vi "Gear Mech Controller.vi"(8 "error in":errorcluster) -> ()   [LabVIEW 2016]
doc: "This VI executes continuously carrying out the current operation and responding to updates or new operations. It will often contain the timing or control code that is difficult to place directly in TeleOp. This VI generally opens all sensors and motors and isolates the rest of the robot code from knowing how the operations are carried out."
uses:
  <vilib>/Rock Robotics/WPI/ThirdParty/CanMotor/TalonSRX/WPI_CANTalonSRX_GlobalStatus.ctl
  Shared/PID Settings.ctl
  Gear Mech Setpoints.ctl
  Gear Mech Operations.ctl
  <vilib>/Rock Robotics/WPI/ThirdParty/CanMotor/TalonSRX/WPI_CANTalonSRX_APIControlMode.ctl
  <vilib>/Rock Robotics/WPI/ThirdParty/CanMotor/TalonSRX/WPI_CANTalonSRX_APIFeedbackSelect.ctl
  <vilib>/Rock Robotics/Network Tables/NT Write Boolean.vi
panel:
  in  "Full Up Position":dbl=600.0
  in  "Boolean":bool
  in  "Shooter PID":T1={"D"=0.01, "F"=0.0, "RR"=0.0, "IZ"=0.0, "P"=3.0, "I"=0.0}
  in  "Down Position":dbl=345.0
  in  "Up Position":dbl=560.0
  in  "In Speed":dbl=0.5
  in  "Out Speed":dbl=-0.5
  out "Talon SRX Status":T2
  out "Current\nCmd":string
  # "Tip: It may be helpful to observe inputs and sensor values.\nYou may also want to display tuning or debugging controls."
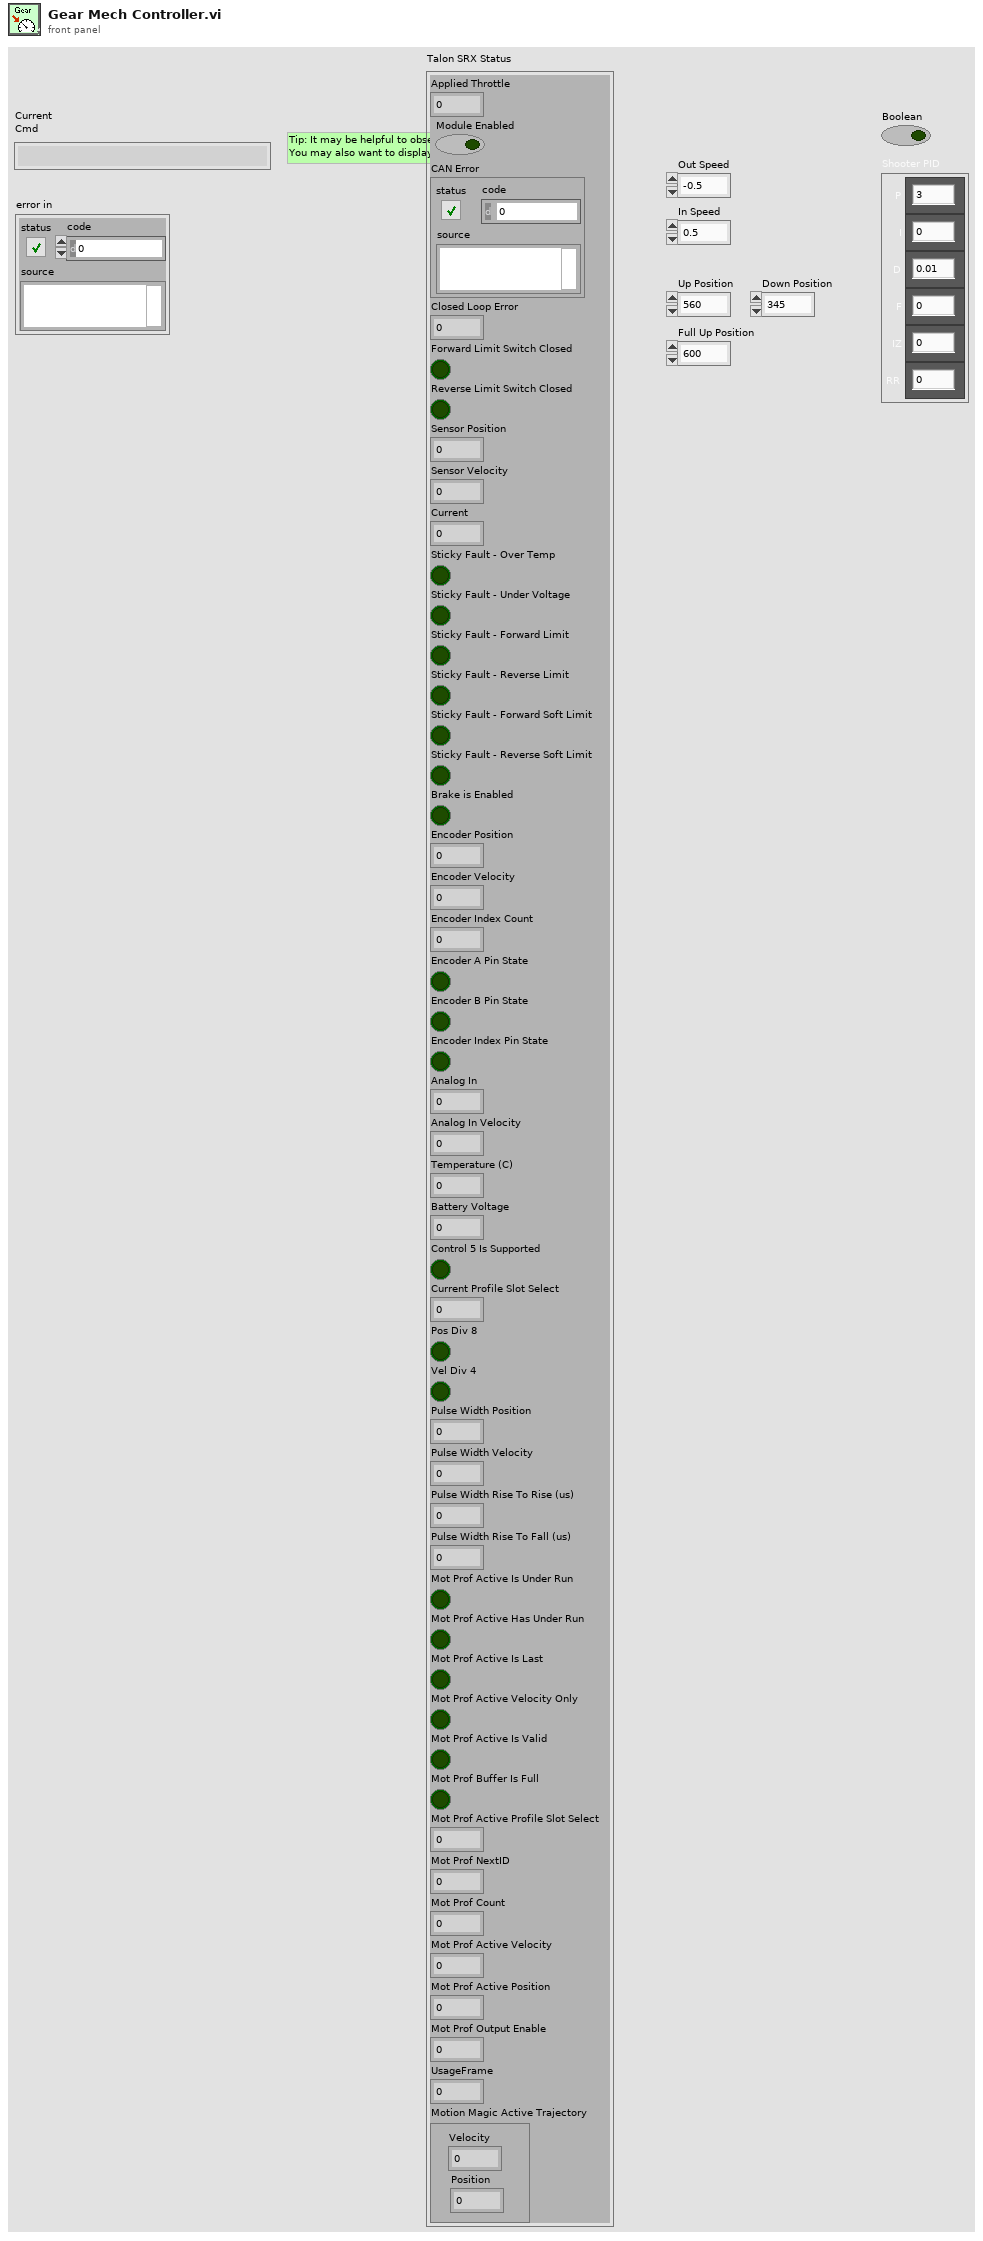
[diagram p1: front panel]
types:
  T1 = typedef "PID Settings.ctl" = cluster{"D":dbl, "F":dbl, "RR":dbl, "IZ":dbl, "P":dbl, "I":dbl}
  T2 = typedef "WPI_CANTalonSRX_GlobalStatus.ctl" = cluster{"Applied Throttle":dbl, "Module Enabled":bool, "CAN Error":errorcluster, "Closed Loop Error":dbl, "Forward Limit Switch Closed":bool, "Reverse Limit Switch Closed":bool, "Sensor Position":dbl, "Sensor Velocity":dbl, "Current":dbl, "Sticky Fault - Over Temp":bool, "Sticky Fault - Under Voltage":bool, "Sticky Fault - Forward Limit":bool, "Sticky Fault - Reverse Limit":bool, "Sticky Fault - Forward Soft Limit":bool, "Sticky Fault - Reverse Soft Limit":bool, "Brake is Enabled":bool, "Encoder Position":dbl, "Encoder Velocity":dbl, "Encoder Index Count":dbl, "Encoder A Pin State":bool, "Encoder B Pin State":bool, "Encoder Index Pin State":bool, "Analog In":dbl, "Analog In Velocity":dbl, "Temperature (C)":dbl, "Battery Voltage":dbl, "Control 5 Is Supported":bool, "Current Profile Slot Select":dbl, "Pos Div 8":bool, "Vel Div 4":bool, "Pulse Width Position":i32, "Pulse Width Velocity":i32, "Pulse Width Rise To Rise (us)":i32, "Pulse Width Rise To Fall (us)":i32, "Mot Prof Active Is Under Run":bool, "Mot Prof Active Has Under Run":bool, "Mot Prof Active Is Last":bool, "Mot Prof Active Velocity Only":bool, "Mot Prof Active Is Valid":bool, "Mot Prof Buffer Is Full":bool, "Mot Prof Active Profile Slot Select":i32, "Mot Prof NextID":i32, "Mot Prof Count":i32, "Mot Prof Active Velocity":dbl, "Mot Prof Active Position":dbl, "Mot Prof Output Enable":i32, "UsageFrame":u32, "Motion Magic Active Trajectory":cluster{"Velocity":dbl, "Position":dbl}}
  T3 = typedef "WPI_CANTalonSRX_APIControlMode.ctl" = enum8{"Percent VBus", "Speed", "Position", "Slave", "Unchanged / Invalid", "Voltage Compensation", "Current", "Motion Profile", "Motion Magic"}
  T4 = typedef "WPI_CANTalonSRX_APIFeedbackSelect.ctl" = enum16{"Digital Quadrature Encoder", "Analog Potentiometer", "Analog Encoder", "Count on Quad-A (Rising-Edge)", "Count on Quad-A (Falling-Edge)", "CTR Magnetic Enc (Absolute)", "CTR Magnetic Enc (Relative)", "Pulse Width"}
  T5 = typedef "Gear Mech Setpoints.ctl" = cluster{"Operation":T6, "Setpoint":dbl, "Duration":dbl}
  T6 = typedef "Gear Mech Operations.ctl" = enum16{"Reserve", "Read Current", "Immediate", "Release", "Grab", "Up", "Down", "Full Up"}
  T7 = typedef "WPI_MotorControlDeviceRef.ctl" = cluster{"DeviceStatus":errorcluster, "Type":T8, "PWM":cluster{"PWM Channel":T9, "DeadBand":T10}, "CAN":cluster{"Device Number":u8, "SetOutput VI Ref":variant, "GetOutput VI Ref":variant, "Enable VI Ref":variant, "Disable VI Ref":variant, "Data":variant}, "Invert":bool}
  T8 = typedef "WPI_MotorControlType.ctl" = enum16{"PWM", "CAN"}
  T9 = typedef "FPGA_DIOPWMChannel.ctl" = enum8{"PWM 0", "PWM 1", "PWM 2", "PWM 3", "PWM 4", "PWM 5", "PWM 6", "PWM 7", "PWM 8", "PWM 9", "PWM MXP 0", "PWM MXP 1", "PWM MXP 2", "PWM MXP 3", "PWM MXP 4", "PWM MXP 5", "PWM MXP 6", "PWM MXP 7", "PWM MXP 8", "PWM MXP 9", "Invalid"}
  T10 = typedef "WPI_PWMDeadband.ctl" = cluster{"Name":string, "maxPositivePwm":i32, "minPositivePwm":i32, "centerPwm":i32, "maxNegativePwm":i32, "minNegativePwm":i32, "angularRange":u16}
  T11 = typedef "Command Status Info.ctl" = cluster{"Name":string, "Status":T12, "notifier out":T13}
  T12 = typedef "Completion Status.ctl" = enum16{"Successful", "Aborted", "Incomplete"}
  T13 = typedef "Completion Notifier.ctl" = refnum<notifier>
  T14 = cluster{"Default Command":T5, "Command Timing":cluster{"Start Time (ms)":u32, "Iterations":i32}, "Command Arguments":cluster{"Command Info":T11, "Description":string, "Default Command":T5, "notifier out":refnum<notifier>, "Subsystem Name":string}}
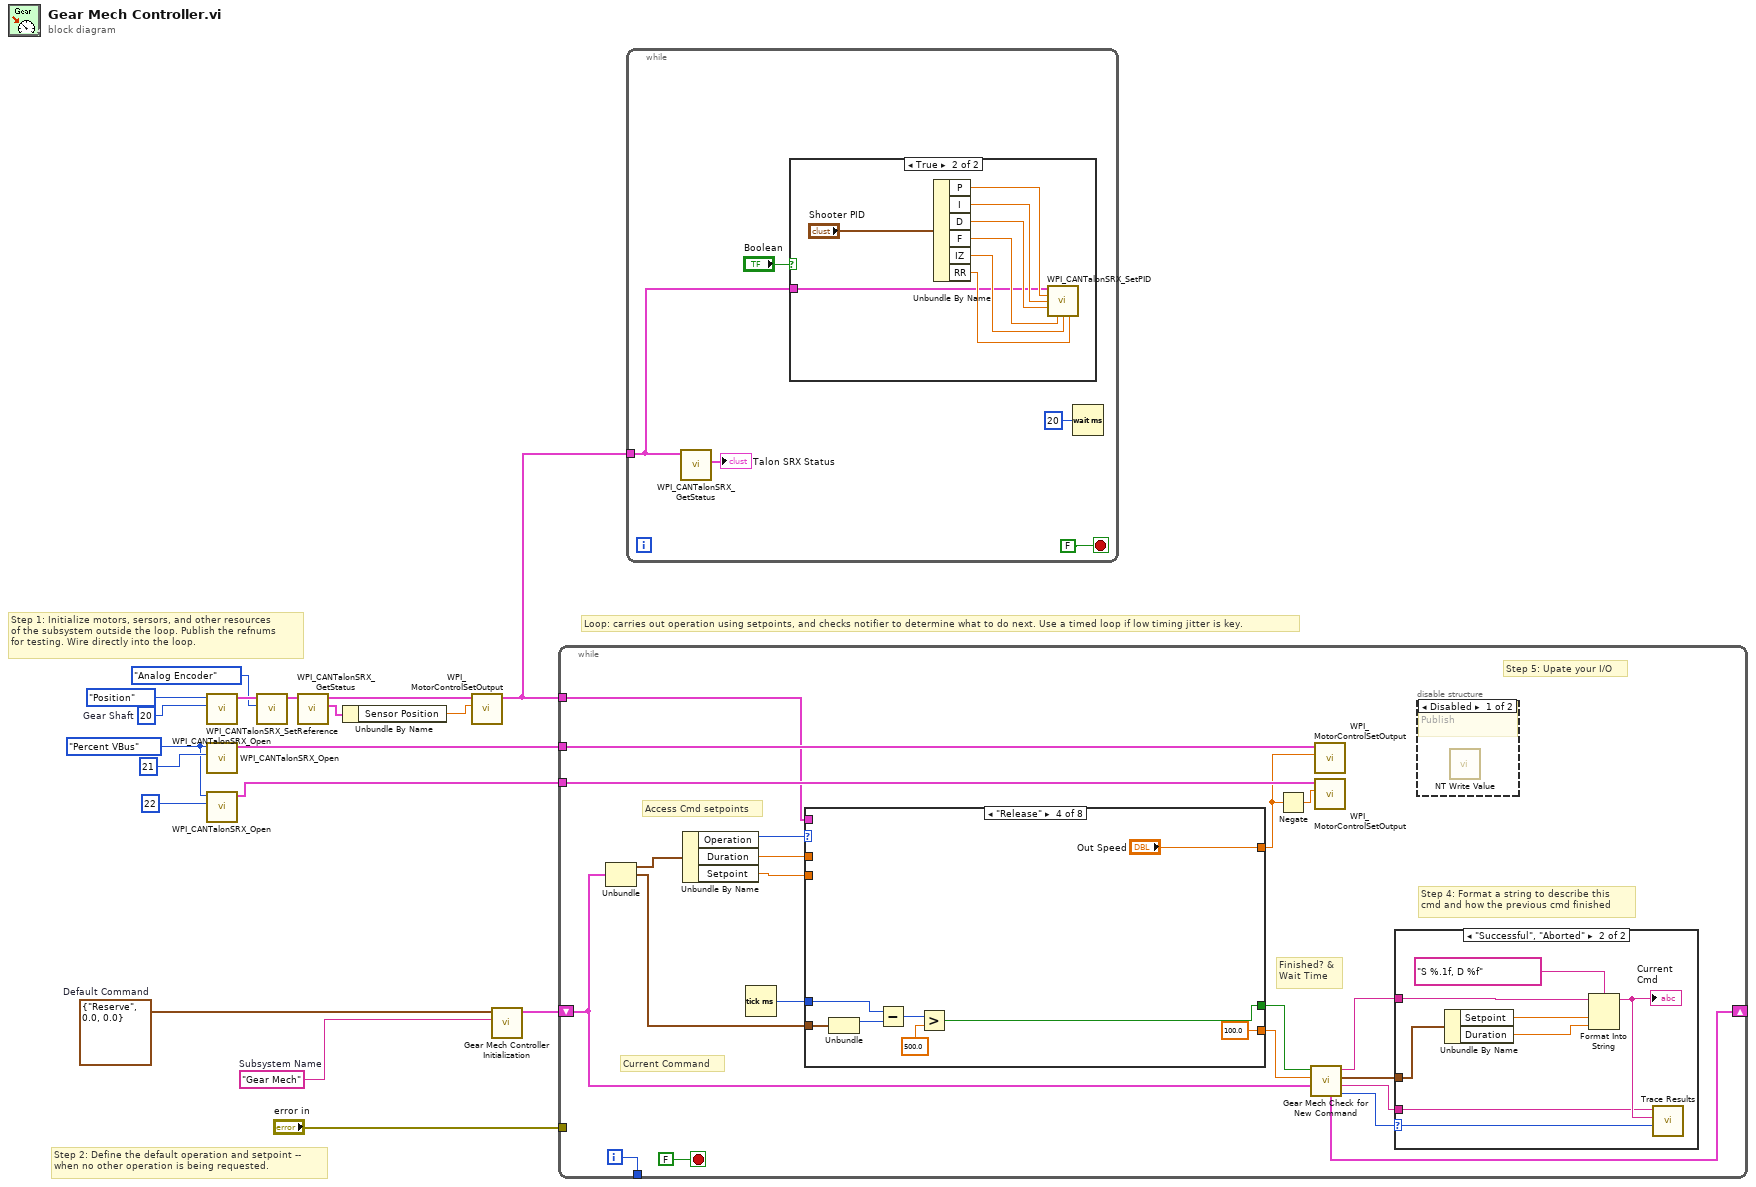
[diagram p0: block diagram]
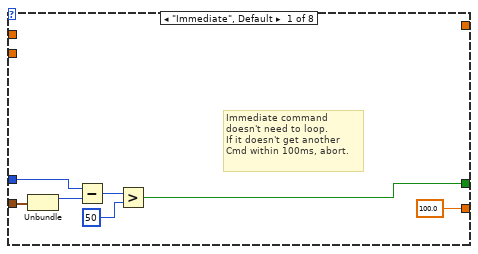
[diagram p5: hidden frame]
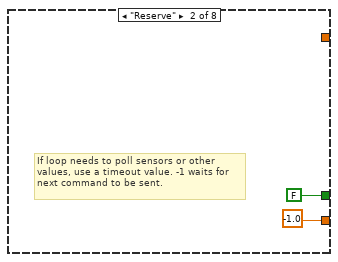
[diagram p6: hidden frame]
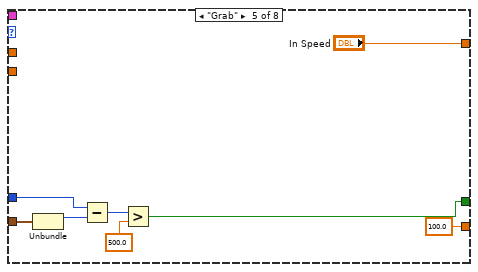
[diagram p8: hidden frame]
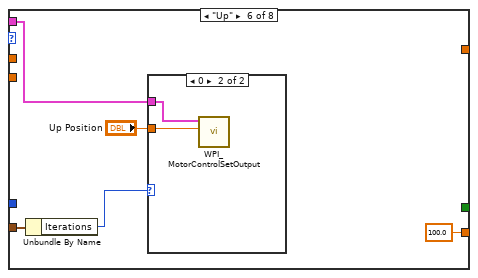
[diagram p9: hidden frame]
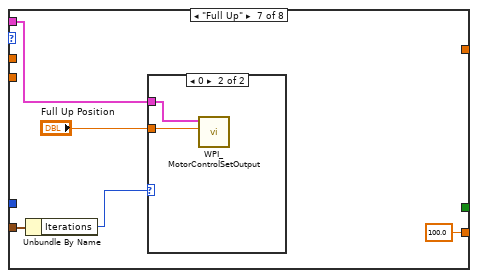
[diagram p11: hidden frame]
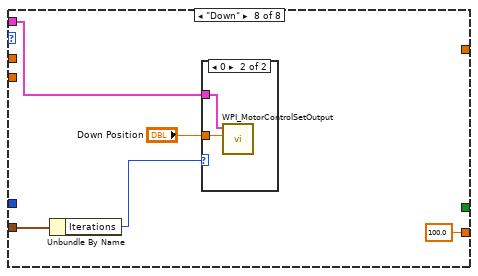
[diagram p13: hidden frame]
diagram:
  w7 = WPI_CANTalonSRX_APIControlMode."Percent VBus" ("Control Mode")
  w13 = u8 20  # Gear Shaft
  w15 = T5 {"Operation"=enum."Reserve", "Setpoint"=0.0, "Duration"=0.0}  # Default Command
  w16 = "Gear Mech"  # Subsystem Name
  # "Step 2: Define the default operation and setpoint --\nwhen no other operation is being requested."
  # "Step 1: Initialize motors, sersors, and other resources\nof the subsystem outside the loop. Publish the refnums\nfor testing. Wire directly into the loop."
  # "Loop: carries out operation using setpoints, and checks notifier to determine what to do next. Use a timed loop if low timing jitter is key."
  n1 = call <vilib>:"WPI_CANTalonSRX_Open.vi"("Device Number"=w13, "Control Mode"=WPI_CANTalonSRX_APIControlMode."Position") -> ("CAN Talon SRX Ref"=w12:T7)  [unwired: 8 in, 1 out]
  n2 = call <vilib>:"WPI_CANTalonSRX_Open.vi"("Device Number"=u8 21, "Control Mode"=w7) -> ("CAN Talon SRX Ref"=w10:T7)  [unwired: 8 in, 1 out]
  n3 = call <vilib>:"WPI_CANTalonSRX_Open.vi"("Device Number"=u8 22, "Control Mode"=w7) -> ("CAN Talon SRX Ref"=w6:T7)  [unwired: 8 in, 1 out]
  n4 = call <vilib>:"WPI_CANTalonSRX_SetReference.vi"("Feedback Reference"=WPI_CANTalonSRX_APIFeedbackSelect."Analog Encoder", "CAN Talon SRX Ref"=w12) -> ("CAN Talon SRX Ref"=w5:T7)  [unwired: 8 in, 1 out]
  n5 = call <vilib>:"WPI_CANTalonSRX_GetStatus.vi"("CAN Talon SRX Ref"=w5) -> ("Talon SRX Status"=w4:T2, "CAN Talon SRX Ref"=w3:T7)  [unwired: 8 in, 1 out]
  n6 = Unbundle By Name(w4) -> ("Sensor Position"=w1:dbl)
  n7 = call <vilib>:"WPI_MotorControlSetOutput.vi"("Output"=w1, "MotorControlDevRef"=w3) -> ("MotorControlDevRef"=w2:T7)  [unwired: 7 in, 2 out]
  n8 = call "Gear Mech Controller Initialization.vi"("Subsystem Name"=w16, "Default Command"=w15) -> ("Command Info"=w17:T14)  [unwired: 9 in]
  n9 = while {
    shift-right: [w30] -> _
    shift-left: w17 -> [w31]
    tunnel: [w38] -> _
    tunnel: "error in" -> [_]
    tunnel: w2 -> [w19]
    tunnel: w10 -> [w23]
    tunnel: w6 -> [w22]
    i -> [w38]
    stop <- FALSE stop-if-true
    # "Step 5: Upate your I/O"
    # "Step 4: Format a string to describe this\ncmd and how the previous cmd finished"
    # "Current Command"
    # "Access Cmd setpoints"
    # "Finished? &\nWait Time"
    n10 = Unbundle(w31) -> ("Default Command"=w37:T5, "Command Timing"=w33:cluster{"Start Time (ms)":u32, "Iterations":i32})  [unwired: 1 out]
    n11 = Unbundle By Name(w37) -> ("Operation"=w36:T6, "Duration"=w35:dbl, "Setpoint"=w32:dbl)
    n12 = Tick Count (ms)() -> (millisecond timer value=w34:u32)
    n13 = case shown="\"Release\"" w36 {
      tunnel: [100.0 -1.0 _ 100.0 100.0 100.0 100.0 100.0] -> w28
      tunnel: [w48 FALSE ("ignore previous (F)") _ w58 w66 _ _ _] -> w29
      tunnel: w33 -> [w50 _ _ w60 w68 w76 w83 w89]
      tunnel: w35 -> [_ _ _ _ _ _ _ _]
      tunnel: w34 -> [w49 _ _ w59 w67 _ _ _]
      tunnel: w32 -> [_ _ _ _ _ _ _ _]
      tunnel: [_ _ _ "Out Speed" "In Speed" _ _ _] -> w21
      tunnel: w19 -> [_ _ _ _ _ w74 w81 w87]
      frame "Immediate", Default {
        # "Immediate command\ndoesn't need to loop.\nIf it doesn't get another\nCmd within 100ms, abort."
        n14 = Unbundle(w50) -> ("Start Time (ms)"=w53:u32)  [unwired: 1 out]
        n15 = Subtract(x=w49, y=w53) -> (x-y=w52:u32)
        n16 = Greater?(x=w52, y=u8 50 ("Left Motor")) -> (0:w48:bool)
      }
      frame "Reserve" {
        # "If loop needs to poll sensors or other\nvalues, use a timeout value. -1 waits for\nnext command to be sent."
      }
      frame "Read Current" {
      }
      frame "Release" {
        n17 = Unbundle(w60) -> ("Start Time (ms)"=w61:u32)  [unwired: 1 out]
        n18 = Subtract(x=w59, y=w61) -> (x-y=w63:u32)
        n19 = Greater?(x=w63, y=500.0 ("Out Time")) -> (0:w58:bool)
      }
      frame "Grab" {
        n20 = Unbundle(w68) -> ("Start Time (ms)"=w69:u32)  [unwired: 1 out]
        n21 = Subtract(x=w67, y=w69) -> (x-y=w71:u32)
        n22 = Greater?(x=w71, y=500.0 ("In Time")) -> (0:w66:bool)
      }
      frame "Up" {
        n23 = Unbundle By Name(w76) -> ("Iterations"=w75:i32)
        n24 = case shown="0" w75 {
          tunnel: w74 -> [_ w79]
          tunnel: "Up Position" -> [_ w78]
          frame Default {
          }
          frame 0 {
            n25 = call <vilib>:"WPI_MotorControlSetOutput.vi"("Output"=w78, "MotorControlDevRef"=w79) -> ()  [unwired: 7 in, 3 out]
          }
        }
      }
      frame "Full Up" {
        n26 = Unbundle By Name(w83) -> ("Iterations"=w82:i32)
        n27 = case shown="0" w82 {
          tunnel: w81 -> [_ w86]
          tunnel: "Full Up Position" -> [_ w85]
          frame Default {
          }
          frame 0 {
            n28 = call <vilib>:"WPI_MotorControlSetOutput.vi"("Output"=w85, "MotorControlDevRef"=w86) -> ()  [unwired: 7 in, 3 out]
          }
        }
      }
      frame "Down" {
        n29 = Unbundle By Name(w89) -> ("Iterations"=w90:i32)
        n30 = case shown="0" w90 {
          tunnel: "Down Position" -> [_ w93]
          tunnel: w87 -> [_ w92]
          frame Default {
          }
          frame 0 {
            n31 = call <vilib>:"WPI_MotorControlSetOutput.vi"("Output"=w93, "MotorControlDevRef"=w92) -> ()  [unwired: 7 in, 3 out]
          }
        }
      }
    }
    n32 = Negate(x=w21) -> (-x=w20:dbl)
    n33 = call "Gear Mech Check for New Command.vi"("Current Command"=w31, "Wait time (ms)"=w28, "Finished?"=w29) -> ("Completion"=w24:T12, "Subsystem Name"=w25:string, "Current Command"=w26:T5, "Initial Trace String"=w27:string, "NextCommand"=w30:T14)  [unwired: 4 in]
    n34 = call <vilib>:"WPI_MotorControlSetOutput.vi"("Output"=w21, "MotorControlDevRef"=w23) -> ()  [unwired: 7 in, 3 out]
    n35 = call <vilib>:"WPI_MotorControlSetOutput.vi"("Output"=w20, "MotorControlDevRef"=w22) -> ()  [unwired: 7 in, 3 out]
    n36 = case shown="\"Successful\", \"Aborted\"" w24 {
      selector: w24 -> [_ w47]
      tunnel: w27 -> [_ w43]
      tunnel: w26 -> [_ w44]
      tunnel: w25 -> [_ w40]
      frame "Incomplete", Default {
        # "Continuing current command"
      }
      frame "Successful", "Aborted" {
        # "Report and setup for next command"
        n37 = Unbundle By Name(w44) -> ("Setpoint"=w46:dbl, "Duration"=w41:dbl)
        n38 = Format Into String(format string="S %.1f, D %f", initial string=w43, w46, w41) -> (resulting string=w42:string)  [unwired: 1 in, 1 out]
        "Current\nCmd" <- w42
        n39 = call <vilib>:"Trace Results.vi"("Status of previous command"=w47, "Description"=w42, "Subsystem"=w40) -> ()  [unwired: 9 in]
      }
    }
    n40 = disable-structure shown="Disabled" {
      frame Disabled {
        # "Publish"
        n41 = call-poly <vilib>:"NT Write Value.vi"() -> ()  [unwired: 11 in, 1 out]
      }
      frame Enabled {
      }
    }
  }
  n42 = while {
    tunnel: w2 -> [w95]
    stop <- FALSE stop-if-true
    n43 = call <vilib>:"WPI_CANTalonSRX_GetStatus.vi"("CAN Talon SRX Ref"=w95) -> ("Talon SRX Status"=→"Talon SRX Status":T2)  [unwired: 8 in, 2 out]
    n44 = case shown="True" "Boolean" {
      tunnel: w95 -> [_ w100]
      frame False {
      }
      frame True {
        n45 = Unbundle By Name("Shooter PID") -> ("P"=w105:dbl, "I"=w104:dbl, "D"=w103:dbl, "F"=w102:dbl, "IZ"=w101:dbl, "RR"=w106:dbl)
        n46 = call <vilib>:"WPI_CANTalonSRX_SetPID.vi"("CAN Talon SRX Ref"=w100, "P"=w105, "I"=w104, "D"=w103, "F"=w102, "I Zone"=w101, "Ramp Rate"=w106) -> ()  [unwired: 7 in, 2 out]
      }
    }
    n47 = Wait (ms)(milliseconds to wait=u32 20) -> ()  [unwired: 1 out]
  }
